vi "get_P.vi"(8 "error in (no error)":errorcluster, 11 "VISA Refnum in":refnum<visa-resource-name>) -> (0 "error out":errorcluster, 2 "P":dbl, 3 "VISA Refnum out":refnum<visa-resource-name>)   [LabVIEW 2018]
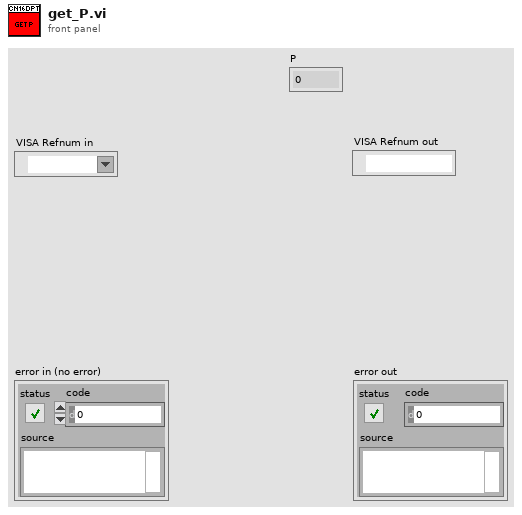
[diagram p1: front panel]
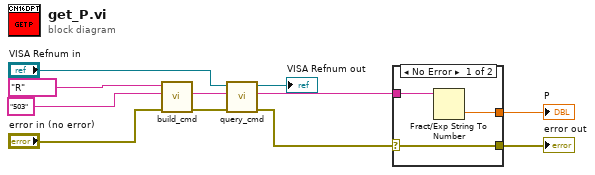
[diagram p0: block diagram]
diagram:
  n1 = call "build_cmd.vi"("error in (no error)"="error in (no error)", "Command ID"="503", "Command class"="R") -> ("error out"=w6:errorcluster, "Command"=w5:string)  [unwired: 7 in]
  n2 = call "query_cmd.vi"("error in (no error)"=w6, "Command"=w5, "VISA resource name"="VISA Refnum in") -> ("error out"=w3:errorcluster, "Response"=w4:string, "VISA resource name out"=→"VISA Refnum out":refnum<visa-resource-name>)  [unwired: 6 in]
  n3 = case shown="No Error" w3 {
    selector: w3 -> [w12 w15]
    tunnel: w4 -> [w14 _]
    tunnel: [w12 w15] -> w2
    tunnel: [w13 _] -> w1
    frame No Error {
      n4 = Fract/Exp String To Number(string=w14) -> (number=w13:dbl)  [unwired: 3 in, 1 out]
    }
    frame Error {
    }
  }
  "error out" <- w2
  "P" <- w1
